vi "UPDATE_VENDING MACHINE.vi"(8 "error in (no error)":errorcluster, 11 "USR":T1) -> (0 "error out":errorcluster)   [LabVIEW 2019, in "DB_VENDING MACHINE.lvlib"]
uses:
  DB_VENDING MACHINE.lvlib
  6 SEMESTRE/ADQUISICION_DATOS/BASE DE DATOS WEB/DB_LIBRARY/USR.ctl
  <vilib>/addons/database/NI_Database_API.lvlib
  6 SEMESTRE/ADQUISICION_DATOS/BASE DE DATOS WEB/DB_LIBRARY/DB_LIBARY.lvlib
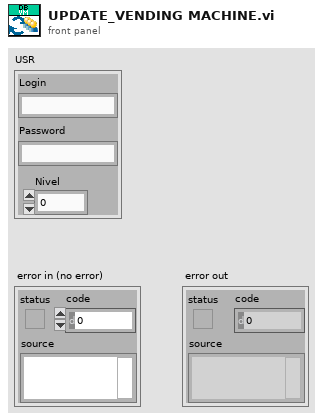
[diagram p1: front panel]
types:
  T1 = typedef "DB_LIBARY.lvlib/USR.ctl" = cluster{"Login":string, "Password":string, "Nivel":u8}
  T2 = typedef "NI_Database_API.lvlib/Conn ObjectReference.ctl" = refnum<k1>
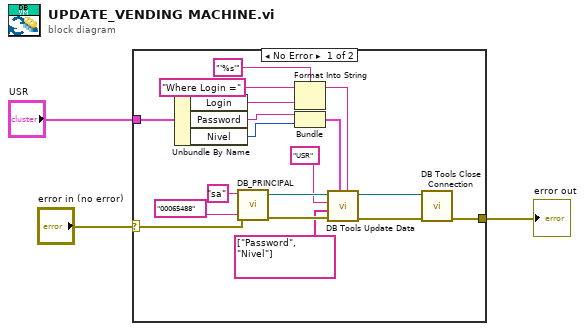
[diagram p0: block diagram]
diagram:
  n1 = case shown="No Error" "error in (no error)" {
    selector: "error in (no error)" -> [w12 w22]
    tunnel: "USR" -> [w7 _]
    tunnel: [w13 w22] -> w2
    frame No Error {
      n2 = Unbundle By Name(w7) -> ("Login"=w9:string, "Password"=w6:string, "Nivel"=w5:u8)
      n3 = call "DB_PRINCIPAL.vi"("error in (no error)"=w12, "password"="00065488", "userID"="sa") -> ("error out"=w20:errorcluster, "connection reference"=w21:T2)  [unwired: 7 in]
      n4 = Format Into String(format string="'%s'", initial string="Where Login =" ("condition"), w9) -> (resulting string=w10:string)  [unwired: 1 in, 1 out]
      n5 = Bundle("Password"=w6, "Nivel"=w5) -> (w8:cluster{"Password":string, "Nivel":u8})  [unwired: 1 in]
      n6 = call <vilib>:"DB Tools Update Data.vi"("condition"=w10, "data"=w8, "error in (no error)"=w20, "columns"=string[] ["Password", "Nivel"], "table"="USR", "connection reference"=w21) -> ("error out"=w19:errorcluster, "connection reference out"=w18:T2)  [unwired: 4 in]
      n7 = call <vilib>:"DB Tools Close Connection.vi"("error in (no error)"=w19, "connection reference"=w18) -> ("error out"=w13:errorcluster)  [unwired: 5 in]
    }
    frame Error {
    }
  }
  "error out" <- w2
